vi "Make_Trail_Array.vi"(10 "Trail_Length":dbl, 11 "Dot_Color":u32(colorbox)) -> (3 "Trail_Array":u32[](array[numeric]))   [LabVIEW 2020]
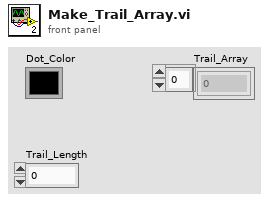
[diagram p1: front panel]
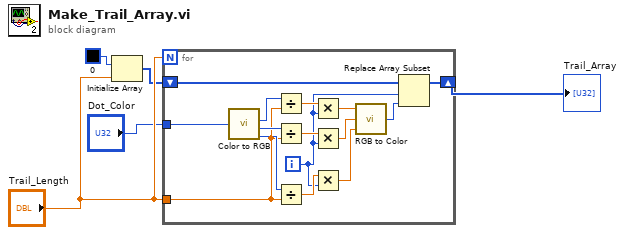
[diagram p0: block diagram]
diagram:
  n1 = Initialize Array(u32 0, "Trail_Length") -> (w1:u32[])
  n2 = for {
    N: "Trail_Length" -> [_]
    tunnel: "Dot_Color" -> [w20]
    tunnel: "Trail_Length" -> [w15]
    shift-right: [w7] -> w4
    shift-left: w1 -> [w6]
    i -> [w8]
    n3 = call <vilib>:"Color to RGB.vi"("Color"=w20) -> ("R"=w19:u8, "G"=w17:u8, "B"=w16:u8)  [unwired: 1 out]
    n4 = Divide(x=w19, y=w15) -> (x/y=w18:dbl)
    n5 = Divide(x=w17, y=w15) -> (x/y=w14:dbl)
    n6 = Divide(x=w16, y=w15) -> (x/y=w13:dbl)
    n7 = Multiply(x=w18, y=w8) -> (x*y=w12:dbl)
    n8 = Multiply(x=w14, y=w8) -> (x*y=w11:dbl)
    n9 = Multiply(x=w13, y=w8) -> (x*y=w10:dbl)
    n10 = call <vilib>:"RGB to Color.vi"("B"=w10, "G"=w11, "R"=w12) -> ("Color"=w9:u32)
    n11 = Replace Array Subset(array=w6, new element=w9, index=w8) -> (w7:u32[])
  }
  "Trail_Array" <- w4
